vi "Read range_AC_check_low_voltage.vi"(8 "error in (no error)":errorcluster, 11 "Report in":refnum<class "Report.lvclass">) -> (0 "error out":errorcluster, 2 "range_AC_check_low_voltage":string[][](table)=[["1", "", "", ""], ["", "", "", ""], ["", "", "", ""], ["", "", "", "4"]], 3 "Report out":refnum<class "Report.lvclass">)   [LabVIEW 2017, in "Report.lvclass"]
uses:
  Report.lvclass
  Report.lvclass/Report.ctl
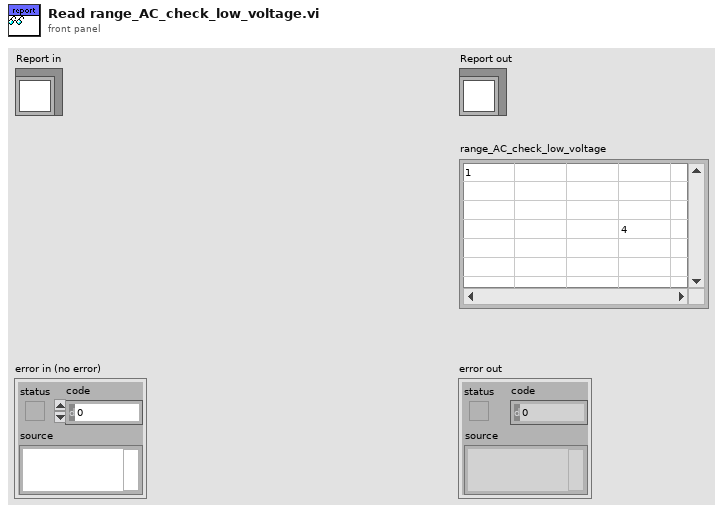
[diagram p1: front panel]
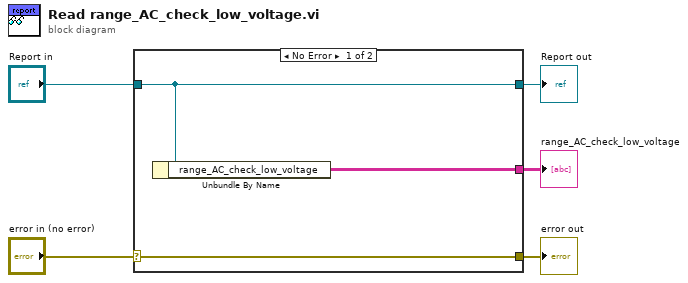
[diagram p0: block diagram]
diagram:
  n1 = case shown="No Error" "error in (no error)" {
    selector: "error in (no error)" -> [w8 w9]
    tunnel: [w8 w9] -> w4
    tunnel: [w7 w10] -> w2
    tunnel: "Report in" -> [w7 w10]
    tunnel: [w6 _] -> w1
    frame No Error {
      n2 = Unbundle By Name(w7) -> ("range_AC_check_low_voltage"=w6:string[][])
    }
    frame Error {
    }
  }
  "error out" <- w4
  "Report out" <- w2
  "range_AC_check_low_voltage" <- w1
